vi "Obtain Control Cluster.vi"(9 "I/O":bool=TRUE, 10 "Dispense":bool=TRUE, 11 "Motion":bool=TRUE) -> (3 "Control Out":T1={"I-O.lvclass"=refnum, "Gantry"=refnum, "Dispenser"="COM1"})   [LabVIEW 2021, in "Controller.lvclass"]
uses:
  Controller.lvclass
  Controllers.ctl
  I-O/I-O.lvclass
  C:/Program Files (x86)/Aerotech/A3200/LabVIEW/2010/Bin/Aerotech.A3200.dll
  Program Files (x86)/Aerotech/A3200/LabVIEW/2010/Bin/Aerotech.A3200.dll
  I-O/NI-DAQ/NI-DAQ.lvclass
  C:/Users/HEP/Documents/GitHub/Gantry/UCSB-Gantry-HEP-main/Classes/Controller/I-O/I-O.lvclass
  Controller.lvclass/Controller.ctl
  Drivers/Aerotech A3200/Aerotech.lvlib
  Drivers/EFD Ultimus V/EFD Ultimus V.lvlib
panel:
  in  "Control":T1={"I-O.lvclass"=refnum, "Gantry"=refnum, "Dispenser"="COM1"}
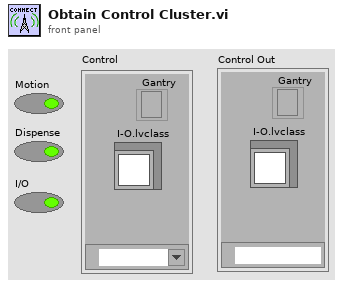
[diagram p1: front panel]
types:
  T1 = typedef "Controller.lvclass/Controllers.ctl" = cluster{"I-O.lvclass":refnum<class "I-O.lvclass">, "Gantry":refnum<k24>, "Dispenser":refnum<visa-resource-name>}
  T2 = typedef "File Paths.ctl" = cluster{"Glue Pattern Folder":path, "Carrier Tray Folder":path, "Pick Up Tool Fixture Folder":path, "Components Folder":path, "Bellows Tool Offset.txt":path, "Pick Up Tool Offset.txt":path, "Dispense Tip Offset.txt":path, "Log Files":path, "Gantry Assembly Map.txt":path, "Syringe and offset map.txt":path, "Controllers Folder":path, "Local dbase config":path}
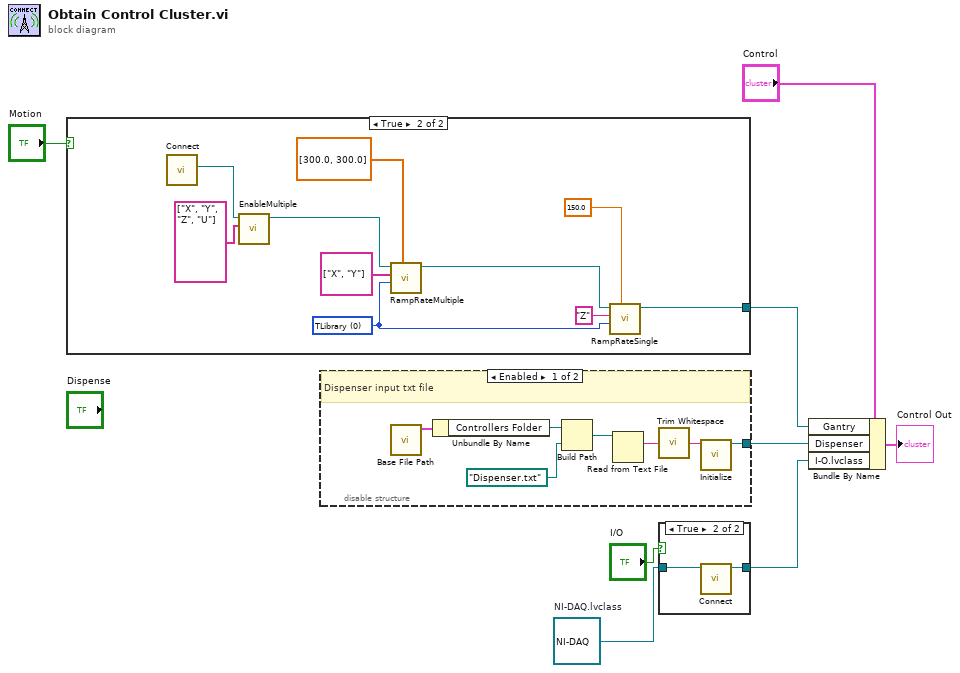
[diagram p0: block diagram]
diagram:
  w4 = refnum<class "NI-DAQ.lvclass"> refnum  # NI-DAQ.lvclass
  n1 = case shown="True" "Motion" {
    tunnel: [_ w10] -> w2
    frame False {
    }
    frame True {
      w11 = 0 items=["TLibrary", "T01", "T02", "T03", "T04", "T05", "T06", "T07", "T08", "T09", "T10", "T11", "T12", "T13", "T14", "T15", "T16", "T17", "T18", "T19", "T20", "T21", "T22", "T23", "T24", "T25", "T26", "T27", "T28", "T29", "T30", "T31"] ("task id")
      n2 = call "Connect.vi"() -> ("controller"=w18:refnum<k24>)  [unwired: 10 in, 1 out]
      n3 = call "EnableMultiple.vi"("axis names"=string[] ["X", "Y", "Z", "U"], "controller in"=w18) -> ("controller out"=w16:refnum<k24>)  [unwired: 8 in, 1 out]
      n4 = call "RampRateMultiple.vi"("ramp rates"=dbl[] [300.0, 300.0], "task id"=w11, "axis names"=string[] ["X", "Y"], "controller in"=w16) -> ("controller out"=w13:refnum<k24>)  [unwired: 6 in, 1 out]
      n5 = call "RampRateSingle.vi"("ramp rate"=150.0, "task id"=w11, "axis name"="Z", "controller in"=w13) -> ("controller out"=w10:refnum<k24>)  [unwired: 6 in, 1 out]
    }
  }
  n6 = disable-structure shown="Enabled" {
    disable-tunnel: [w25 _] -> w1
    frame Enabled {
      # "Dispenser input txt file"
      n7 = call "Base File Path.vi"() -> ("Paths Out"=w24:T2)  [unwired: 11 in]
      n8 = Unbundle By Name(w24) -> ("Controllers Folder"=w23:path)
      n9 = Build Path(base path=w23, name or relative path=path "Dispenser.txt") -> (appended path=w21:path)
      n10 = Read from Text File(file (use dialog)=w21) -> (text=w20:string)  [unwired: 3 in, 3 out]
      n11 = call <vilib>:"Trim Whitespace.vi"("string"=w20) -> ("trimmed string"=w19:string)  [unwired: 1 in]
      n12 = call "Initialize.vi"("VISA resource name"=w19) -> ("VISA resource name out"=w25:refnum<visa-resource-name>)  [unwired: 9 in, 1 out]
    }
    frame Disabled {
    }
  }
  n13 = case shown="True" "I/O" {
    tunnel: w4 -> [w26 w28]
    tunnel: [w26 w27] -> w6
    frame False {
    }
    frame True {
      n14 = call-dynamic "Connect.vi"("NI-DAQ in"=w28) -> ("NI-DAQ out"=w27:refnum<class "NI-DAQ.lvclass">)  [unwired: 9 in, 1 out]
    }
  }
  n15 = Bundle By Name(cluster="Control", "Gantry"=w2, "Dispenser"=w1, "I-O.lvclass"=w6) -> (→"Control Out":T1)
